vi "Process.vi"(8 "error in (no error)":errorcluster, 11 "Icon Decorator In":refnum<class "Icon Decorator.lvclass">) -> (0 "error out":errorcluster, 3 "Icon Decorator Out":refnum<class "Icon Decorator.lvclass">)   [LabVIEW 2020, in "Icon Decorator.lvclass"]
uses:
  Icon Decorator.lvclass
  C:/Git/astemes-lunit/source/Application Framework/Process Classes/Process/Process.lvclass
  Application Framework/Process Classes/Process/Process.lvclass/Process.ctl
  Result Types/Method Result/Method Result type.ctl
  Result Types/Assertion Result/Public/TypeDefs/Status.ctl
  Result Types/Assertion Result/Assertion Result type.ctl
  Result Types/Assertion Result/Public/TypeDefs/Assertion Type.ctl
  Result Types/Case Result/Test Case Result type.ctl
  Result Types/Suite Results/Test Suite Result type.ctl
  Icon Decorator.lvclass/Icon Decorator.ctl
  Application Framework/Process Classes/Process/Public/Accessors/Read Process Name.vi
  <vilib>/Utility/error.llb/Error Cluster From Error Code.vi
  Application Framework/Process Classes/Error Handler/Private/SubVIs/Get Error Queue Name.vi
  <vilib>/ErrorRing/Error Ring.xnode
  Application Framework/Process Classes/Process/Process.lvclass
  Application Framework/Process Classes/Error Handler/Error Handler.lvclass
  Result Types/Assertion Result/Assertion Result.lvlib
  Result Types/Method Result/Method Result.lvlib
  Result Types/Case Result/Test Case Result.lvlib
  Result Types/Suite Results/Test Suite Result.lvlib
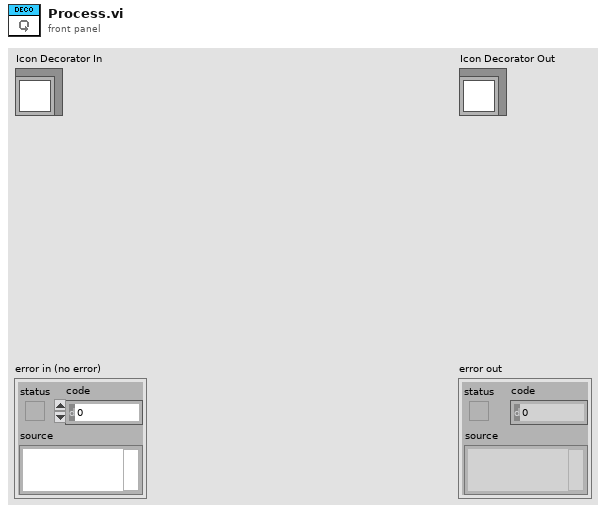
[diagram p1: front panel]
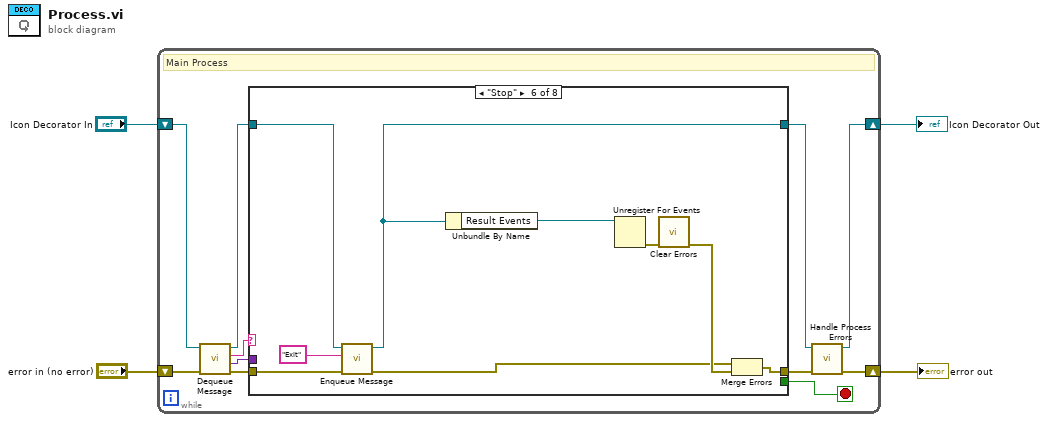
[diagram p0: block diagram]
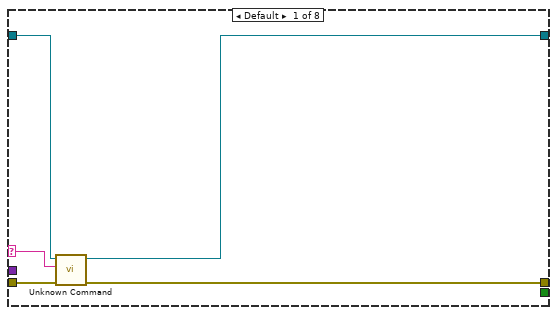
[diagram p2: hidden frame]
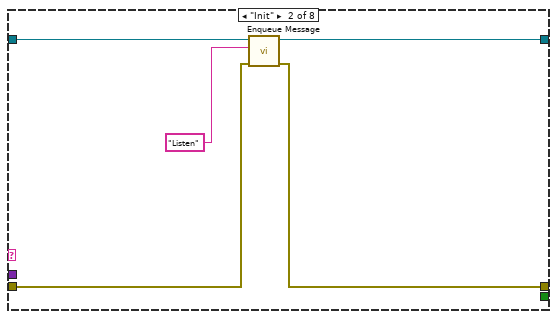
[diagram p3: hidden frame]
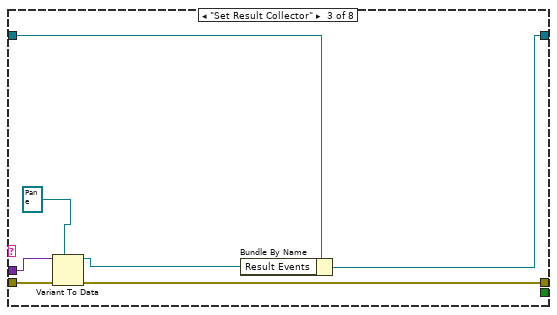
[diagram p4: hidden frame]
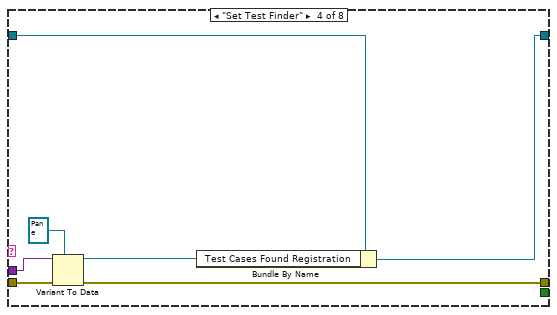
[diagram p5: hidden frame]
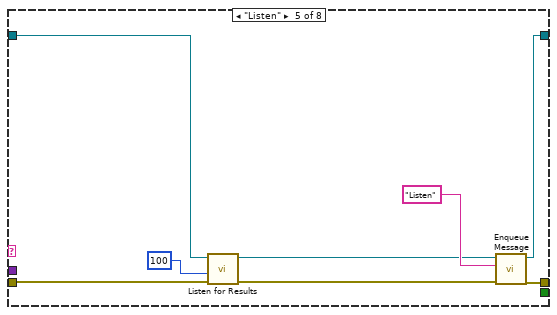
[diagram p6: hidden frame]
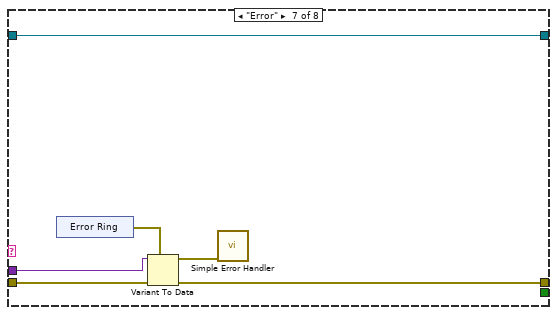
[diagram p7: hidden frame]
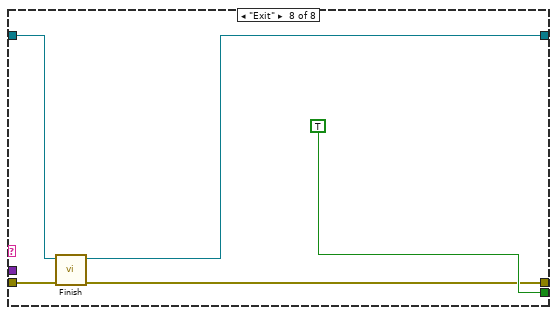
[diagram p8: hidden frame]
diagram:
  n1 = while {
    shift-right: [w7] -> w4
    shift-left: "error in (no error)" -> [w14]
    shift-right: [w5] -> w3
    shift-left: "Icon Decorator In" -> [w15]
    stop <- w9 stop-if-true
    # "Main Process"
    n2 = call "Dequeue Message.vi"("error in (no error)"=w14, "Process In"=w15) -> ("error out"=w13:errorcluster, "Message Data"=w10:variant, "Message"=w11:string, "Process Out"=w12:refnum<class "Icon Decorator.lvclass">)  [unwired: 6 in]
    n3 = case shown="\"Stop\"" w11 {
      selector: w11 -> [w20 _ _ _ _ _ _ _]
      tunnel: [w17 w22 w28 w35 w47 w49 w58 w65] -> w8
      tunnel: w13 -> [w16 w21 w31 w38 w41 w54 w61 w64]
      tunnel: [w19 w24 w29 w36 w46 w53 w62 w66] -> w6
      tunnel: w12 -> [w18 w23 w32 w39 w43 w55 w62 w67]
      tunnel: w10 -> [_ _ w30 w37 _ _ w60 _]
      tunnel: [_ _ _ _ _ _ _ TRUE] -> w9
      frame Default {
        n4 = call "Unknown Command.vi"("error in (no error)"=w16, "String"=w20, "Process In"=w18) -> ("error out"=w17:errorcluster, "Process Out"=w19:refnum<class "Icon Decorator.lvclass">)  [unwired: 7 in]
      }
      frame "Init" {
        n5 = call "Enqueue Message.vi"("error in (no error)"=w21, "Message"="Listen", "Process In"=w23) -> ("error out"=w22:errorcluster, "Process Out"=w24:refnum<class "Icon Decorator.lvclass">)  [unwired: 7 in]
      }
      frame "Set Result Collector" {
        n6 = Variant To Data(error in=w31, type=refnum<event-registration> refnum ("Result Events"), Variant=w30) -> (data=w26:refnum<event-registration>, error out=w28:errorcluster)
        n7 = Bundle By Name(cluster=w32, "Result Events"=w26) -> (w29:refnum<class "Icon Decorator.lvclass">)
      }
      frame "Set Test Finder" {
        n8 = Variant To Data(error in=w38, type=refnum<event-registration> refnum ("Test Cases Found Registration"), Variant=w37) -> (data=w33:refnum<event-registration>, error out=w35:errorcluster)
        n9 = Bundle By Name(cluster=w39, "Test Cases Found Registration"=w33) -> (w36:refnum<class "Icon Decorator.lvclass">)
      }
      frame "Listen" {
        n10 = call "Listen for Results.vi"("error in (no error)"=w41, "Timeout [ms]"=100, "Icon Decorator In"=w43) -> ("error out"=w42:errorcluster, "Icon Decorator Out"=w44:refnum<class "Icon Decorator.lvclass">)  [unwired: 7 in]
        n11 = call "Enqueue Message.vi"("error in (no error)"=w42, "Message"="Listen", "Process In"=w44) -> ("error out"=w47:errorcluster, "Process Out"=w46:refnum<class "Icon Decorator.lvclass">)  [unwired: 7 in]
      }
      frame "Stop" {
        n12 = call "Enqueue Message.vi"("error in (no error)"=w54, "Message"="Exit", "Process In"=w55) -> ("error out"=w48:errorcluster, "Process Out"=w53:refnum<class "Icon Decorator.lvclass">)  [unwired: 7 in]
        n13 = Unbundle By Name(w53) -> ("Result Events"=w52:refnum<event-registration>)
        n14 = Unregister For Events(event registration refnum=w52) -> (error out=w51:errorcluster)  [unwired: 1 in]
        n15 = call <vilib>:"Clear Errors.vi"("error in (no error)"=w51) -> ("error out"=w50:errorcluster)  [unwired: 5 in, 1 out]
        n16 = Merge Errors(w48, w50) -> (w49:errorcluster)
      }
      frame "Error" {
        n17 = xnode "Error Ring"() -> ("error out"=w59:errorcluster)
        n18 = Variant To Data(error in=w61, type=w59, Variant=w60) -> (data=w57:errorcluster, error out=w58:errorcluster)
        n19 = call <vilib>:"Simple Error Handler.vi"("error in (no error)"=w57) -> ()  [unwired: 4 in, 5 out]
      }
      frame "Exit" {
        n20 = call "Finish.vi"("error in (no error)"=w64, "Process In"=w67) -> ("error out"=w65:errorcluster, "Process Out"=w66:refnum<class "Icon Decorator.lvclass">)  [unwired: 8 in]
      }
    }
    n21 = call "Handle Process Errors.vi"("error in (no error)"=w8, "Process In"=w6) -> ("error out"=w7:errorcluster, "Process Out"=w5:refnum<class "Icon Decorator.lvclass">)  [unwired: 8 in]
  }
  "error out" <- w4
  "Icon Decorator Out" <- w3
